vi "MTMount_waitForCompletion_setValue.vi"(8 "error in (no error)":errorcluster, 11 "waitComplete_Ctl":cluster{"cmdSeqNum":i32, "timeout":u32}) -> (0 "error out":errorcluster, 2 "function return":i32, 3 "waitComplete_Ctl out":cluster{"cmdSeqNum":i32, "timeout":u32})   [LabVIEW 2018, in "SALLV_MTMount.lvlib"]
doc: "int MTMount_shm_waitForCompletion_setValueLV(MTMount_waitCompleteLV *waitComplete_Ctl);"
uses:
  SALLV_MTMount.lvlib
  SALLV_MTMount.so
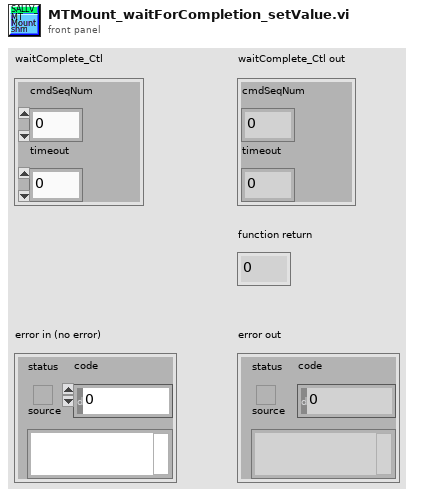
[diagram p1: front panel]
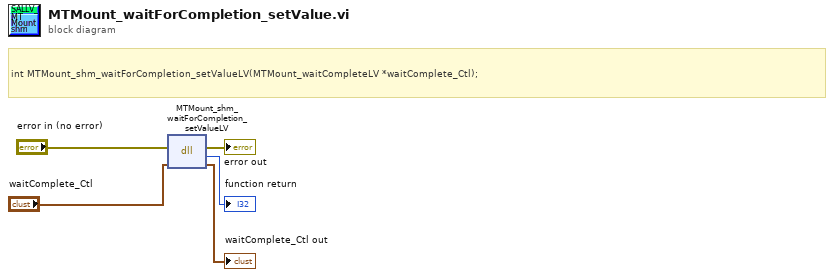
[diagram p0: block diagram]
diagram:
  # "int MTMount_shm_waitForCompletion_setValueLV(MTMount_waitCompleteLV *waitComplete_Ctl);"
  n1 = dll-call lib="home/ttsai/Document/salApiMTMount/SALLV_MTMount/SALLV_MTMount.*" fn="MTMount_shm_waitForCompletion_setValueLV"(error in="error in (no error)", "waitComplete_Ctl"="waitComplete_Ctl") -> (error out=→"error out":errorcluster, →"function return":i32, "waitComplete_Ctl"=→"waitComplete_Ctl out":cluster{"cmdSeqNum":i32, "timeout":u32})  [unwired: 2 in, 1 out]
